vi "load_panel.vi"() -> ()   [LabVIEW 2019]
uses:
  imaginary_stage/subVIs/init_parameters.vi
  ESP301_via_TCPIP/subVIs/init_parameters.vi
  imaginary_stage/imaginaryStage.lvclass
  ESP301_via_TCPIP/ESP301_via_TCPIP.lvclass
panel:
  out "Control Value:Get All":cluster{"Name":string, "Variant Data":variant}[](array[cluster])
  in  "continue":bool
  in  "Enum":enum16{"dummy stage", "ESP301 via TCP/IP"}(ring)
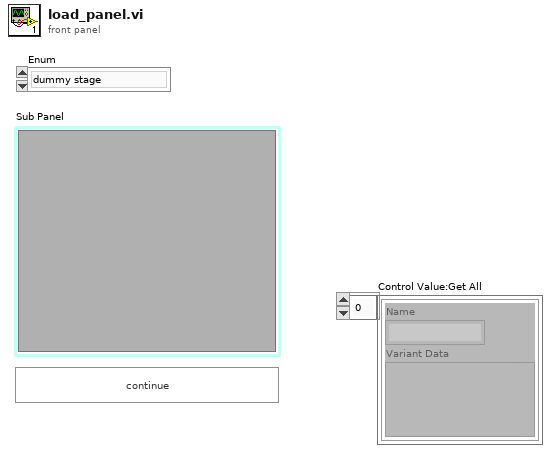
[diagram p1: front panel]
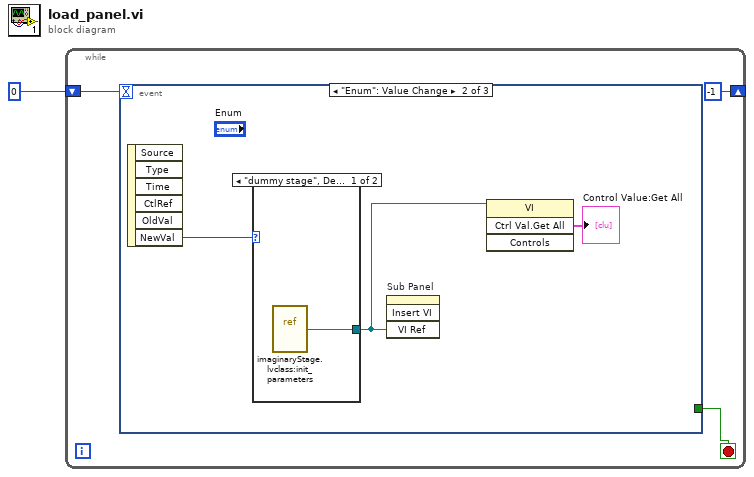
[diagram p0: block diagram]
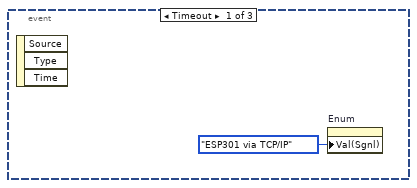
[diagram p2: hidden frame]
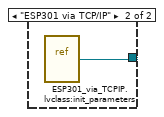
[diagram p3: hidden frame]
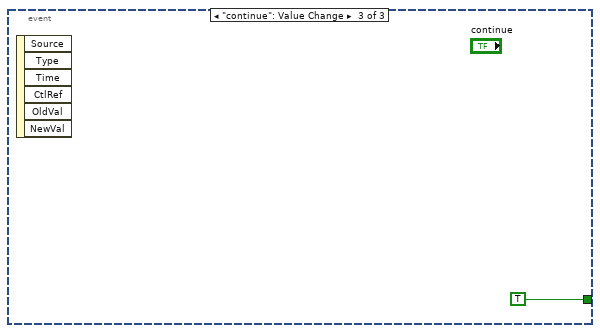
[diagram p4: hidden frame]
diagram:
  n1 = while {
    shift-right: [-1] -> _
    shift-left: 0 -> [w3]
    stop <- w4 stop-if-true
    n2 = event shown="[1] \"Enum\": Value Change" {
      selector: _ -> [_ _ _]
      dyn-events: _ -> [_ _ _]
      timeout: w3 -> [_ _ _]
      tunnel: [_ _ TRUE] -> w4
      event Timeout {
        n3 = event-data() -> ()  [unwired: 1 in, 3 out]
        n4 = property on="Enum" class="Enum (strict)"("Val(Sgnl)"=enum16{"dummy stage", "ESP301 via TCP/IP"}."ESP301 via TCP/IP" ("Value (Signaling)")) -> ()  [unwired: 2 in, 2 out]
      }
      event "Enum": Value Change {
        n5 = event-data() -> ("NewVal"=w8:enum16{"dummy stage", "ESP301 via TCP/IP"})  [unwired: 1 in, 5 out]
        n6 = case shown="\"dummy stage\", Default" w8 {
          tunnel: [w9 w10] -> w7
          frame "dummy stage", Default {
            n7 = vi-ref "imaginaryStage.lvclass:init_parameters.vi"() -> (w9:refnum<vi>)
          }
          frame "ESP301 via TCP/IP" {
            n8 = vi-ref "ESP301_via_TCPIP.lvclass:init_parameters.vi"() -> (w10:refnum<vi>)
          }
        }
        n9 = invoke on="Sub Panel" class="SubPnl" method="Insert VI"("VI Ref"=w7) -> ()  [unwired: 3 in, 4 out]
        n10 = invoke class="VI" method="Ctrl Val.Get All"(reference=w7) -> ("Get All Control Values Variant"=→"Control Value:Get All":cluster{"Name":string, "Variant Data":variant}[])  [unwired: 3 in, 3 out]
      }
      event "continue": Value Change {
        n11 = event-data() -> ()  [unwired: 1 in, 6 out]
      }
    }
  }
